vi "Pre Launch Init.vi"(11 "object in":refnum<class "Actor1_BasicNoLib_N_4.0.0.lvclass">) -> (0 "error out":errorcluster, 3 "object out":refnum<class "Actor1_BasicNoLib_N_4.0.0.lvclass">)   [LabVIEW 2020, in "Actor1_BasicNoLib_N_4.0.0.lvclass"]
uses:
  <resource>/Framework/Providers/Open_GDS/ClassProviders/ActorFramework/4.0.0/Actor1_BasicNoLib_N_4.0.0/Actor1_BasicNoLib_N_4.0.0_class/Actor1_BasicNoLib_N_4.0.0.lvclass
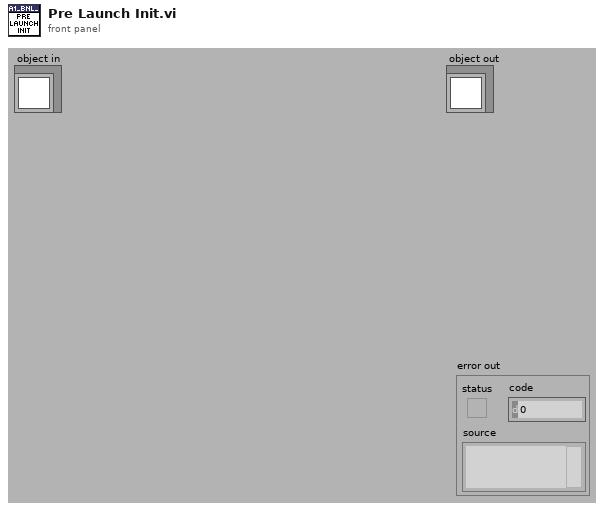
[diagram p1: front panel]
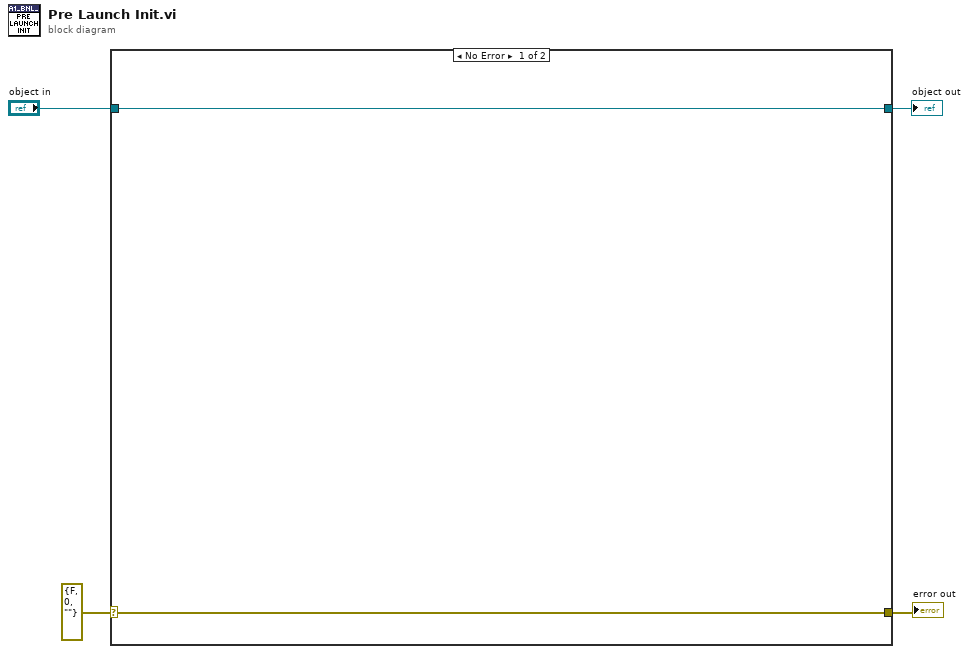
[diagram p0: block diagram]
diagram:
  n1 = case shown="No Error" errorcluster {"status"=FALSE, "code"=0, "source"=""} ("error in (no error)") {
    selector: errorcluster {"status"=FALSE, "code"=0, "source"=""} ("error in (no error)") -> [w6 w8]
    tunnel: [w6 w8] -> w3
    tunnel: [w5 w7] -> w1
    tunnel: "object in" -> [w5 w7]
    frame No Error {
    }
    frame Error {
    }
  }
  "error out" <- w3
  "object out" <- w1
